vi "configure operation.vi"(7 "tag bus configurable plugin module configuration":refnum<class "Modbus Slave configuration.lvclass">, 8 "error in":errorcluster, 10 "line item in":T2, 11 "engine configuration":refnum<class "engine configuration.lvclass">) -> (0 "error out":errorcluster, 1 "success":bool, 2 "line item out":T2, 5 "changed":bool)   [LabVIEW 2013, in "Modbus Slave editor node.lvclass"]
doc: "Platypus Framework 1.0.1.65\nNI Systems Engineering - National Instruments"
uses:
  Modbus Slave editor node.lvclass
  permissions.ctl
  table line.ctl
  module/module channel/Modbus Module Channel.lvclass
  <vilib>/NI/Module Execution Interface/Engine Configuration/engine configuration.lvclass
  module/configuration/Modbus Slave configuration.lvclass
  module/module channel/data bank type.ctl
  <vilib>/NI/Tag Bus Module Framework/channel/TBM channel.lvclass/TBM channel.ctl
  module/module channel/Modbus Module Channel.lvclass/Modbus Module Channel.ctl
  <vilib>/NI/Tag Bus/tag/tag descriptor.lvclass/tag descriptor.ctl
  <vilib>/NI/Configuration Framework/serializable configuration/NISE_CEF_serializable configuration.lvclass/NISE_CEF_serializable configuration.ctl
  <vilib>/NI/Configuration Framework/serializable configuration/NISE_CEF_serializable configuration.lvclass
  <vilib>/NI/Tag Bus/tag/Data Type.ctl
  <vilib>/NI/Tag Bus Module Framework/channel/Read channel classification.vi
  module/module channel/Read modbus type.vi
  module/module channel/Read starting address.vi
  module/module channel/Read subindex (bool).vi
  <vilib>/NI/Tag Bus/tag/read data type.vi
  <vilib>/NI/Configuration Framework/serializable configuration/Read UID.vi
  <vilib>/NI/Tag Bus/tag/write data type.vi
  <vilib>/NI/Tag Bus Module Framework/channel/Write channel classification.vi
  module/module channel/Write modbus type.vi
  module/module channel/Write starting address.vi
  module/module channel/Write subindex (bool).vi
  <vilib>/NI/Tag Bus/tag/write tag name.vi
  <vilib>/NI/Tag Bus/tag/tag descriptor.lvclass
panel:
  in  "Channel Name":string
  out "Alias":string
  out "issues":string
  in  "Tag":i32(listbox)
  in  "Type":i32(listbox)
  in  "Bit":i32 min=0 max=15 step=1
  in  "Address (0 index)":i32
  in  "modbus bank":T1
  in  "cancel":bool
  in  "ok":bool
  in  "Access Type":T3
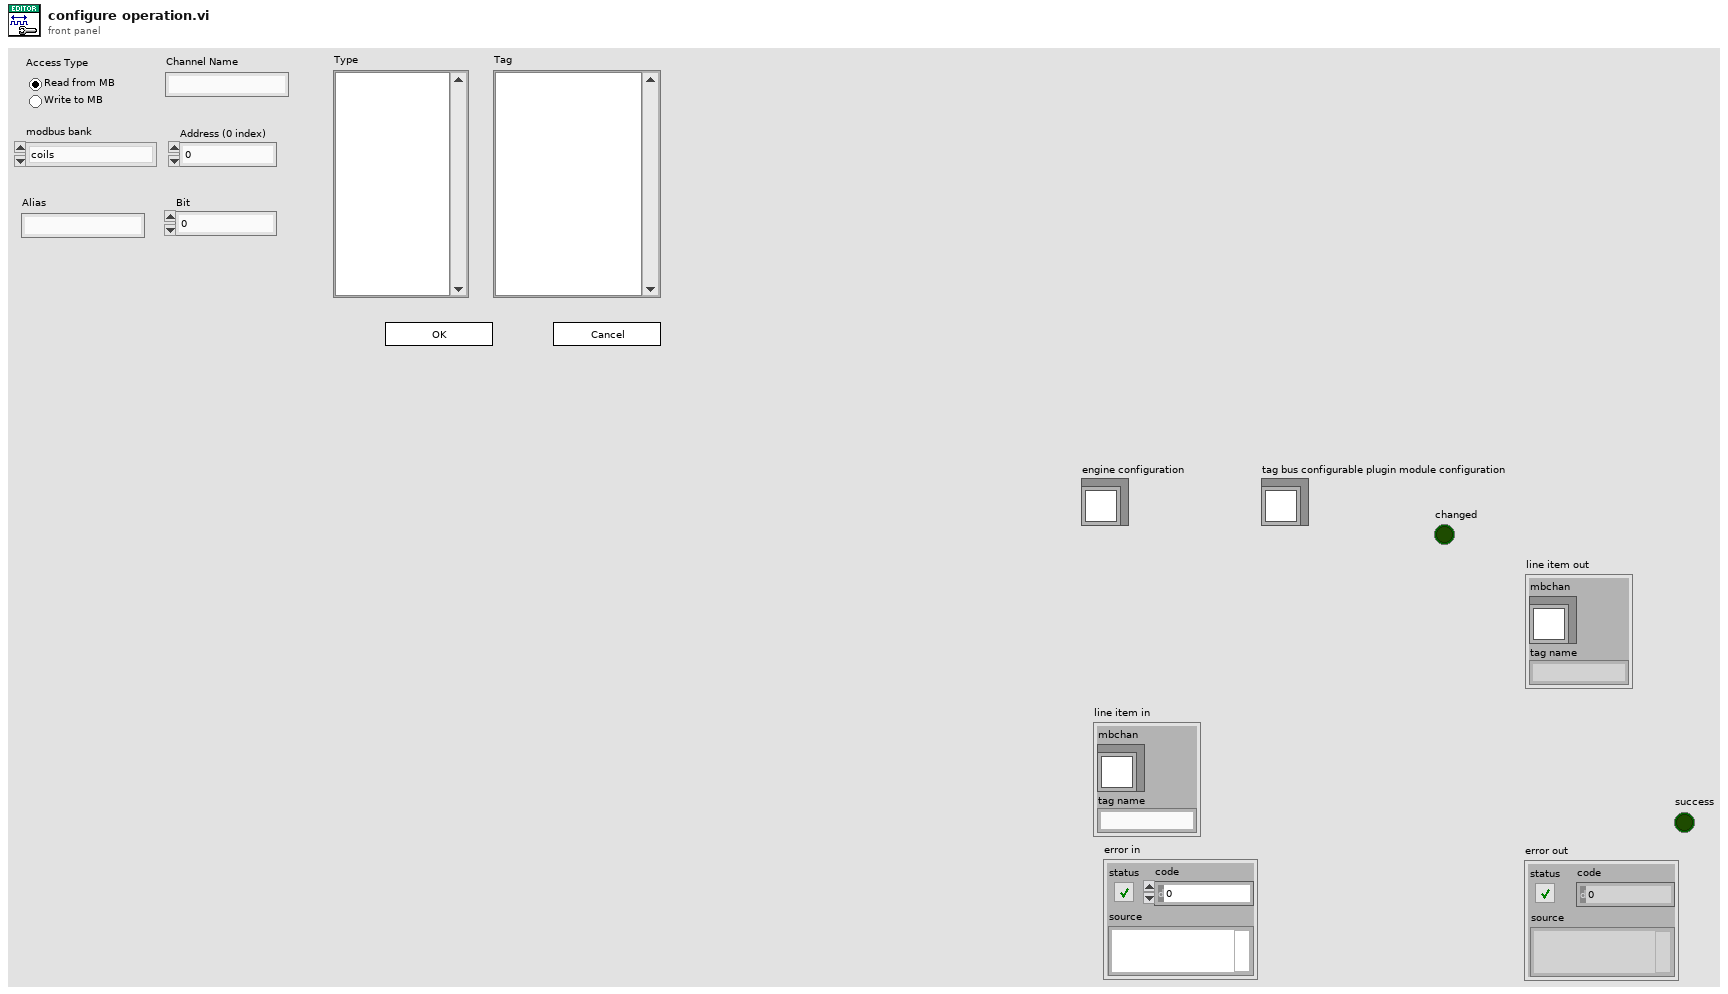
[diagram p1: front panel]
types:
  T1 = typedef "Modbus Module Channel.lvclass/data bank type.ctl" = enum16{"coils", "discrete inputs", "input registers", "holding registers"}
  T2 = typedef "Modbus Slave editor node.lvclass/table line.ctl" = cluster{"mbchan":refnum<class "Modbus Module Channel.lvclass">, "tag name":string}
  T3 = typedef "Modbus Slave editor node.lvclass/permissions.ctl" = enum32{"Read from MB", "Write to MB"}
  T4 = enum32{"Invalid", "Standard", "Closed", "Hidden", "Minimized", "Maximized"}
  T5 = enum32{"Invalid", "Default", "Floating", "Floating/Auto-Hide", "Modal"}
  T6 = enum8{"Enabled", "Disabled", "Disabled and Grayed Out"}
  T7 = typedef "tag bus.lvlib/tag descriptor.lvclass/Data Type.ctl" = enum16{"Double", "Single", "I64", "I32", "I16", "I8", "U64", "U32", "U16", "U8", "Boolean", "String", "Array of Double", "Array of Single", "Array of I64", "Array of I32", "Array of I16", "Array of I8", "Array of U64", "Array of U32", "Array of U16", "Array of U8", "Array of Boolean", "Array of String"}
  T8 = enum32{"invalid app kind", "Development System", "Run Time System", "Student Edition", "Embedded LabVIEW", "Evaluation", "Custom"}
  T9 = typedef "TBM channel.lvclass/channel classification.ctl" = enum16{"input data", "output data", "processing parameter", "processing result"}
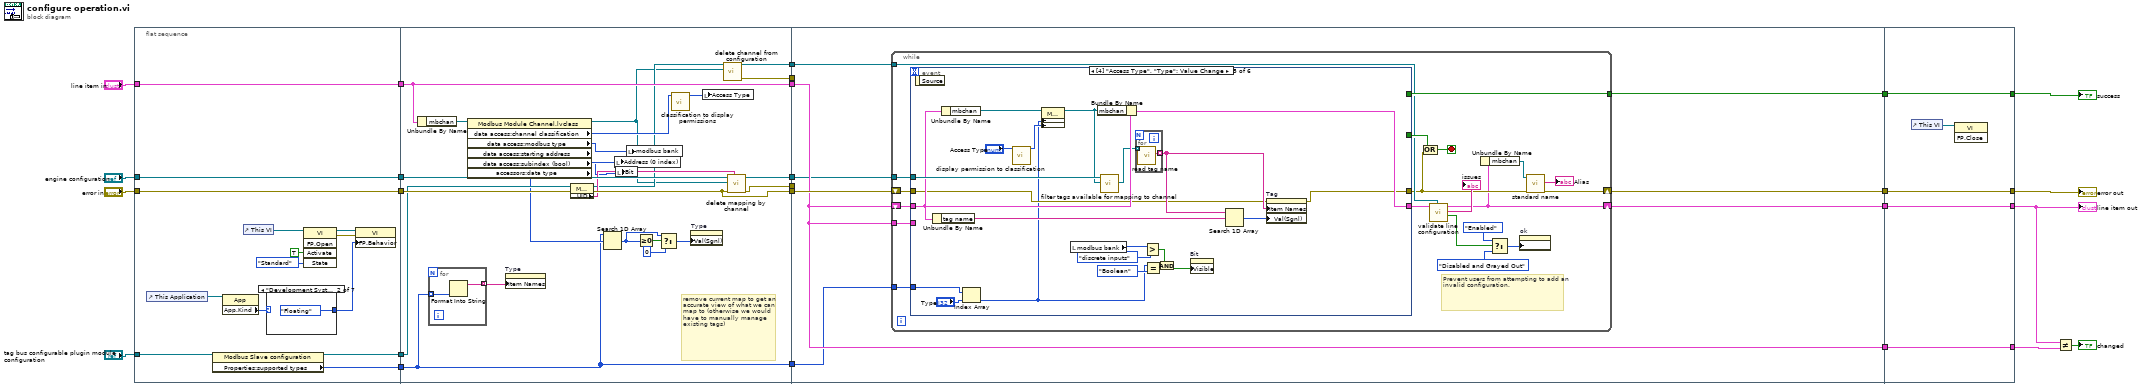
[diagram p0: block diagram]
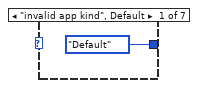
[diagram p2: hidden frame]
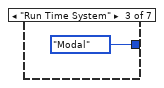
[diagram p3: hidden frame]
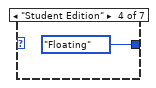
[diagram p4: hidden frame]
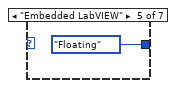
[diagram p5: hidden frame]
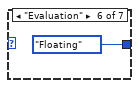
[diagram p6: hidden frame]
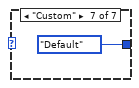
[diagram p7: hidden frame]
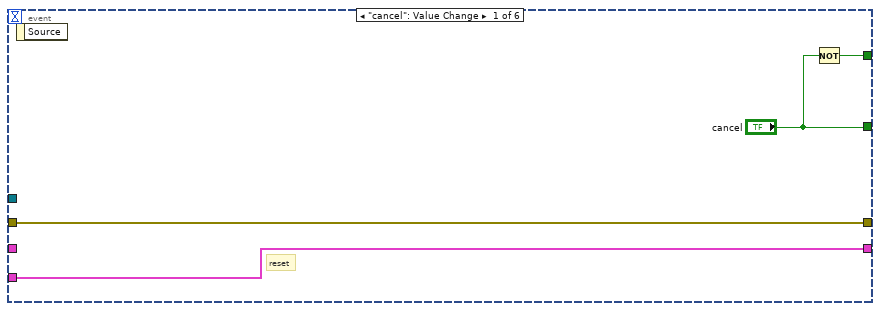
[diagram p8: hidden frame]
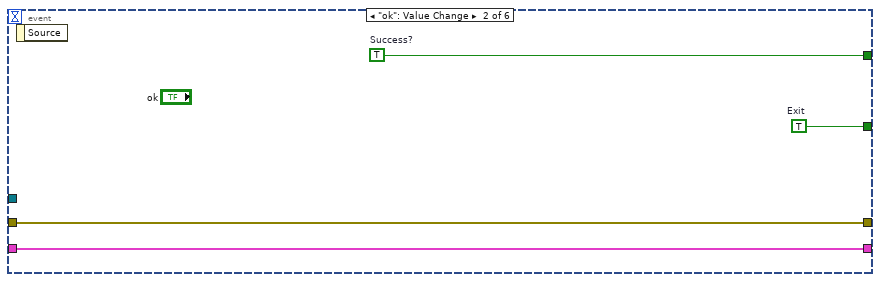
[diagram p9: hidden frame]
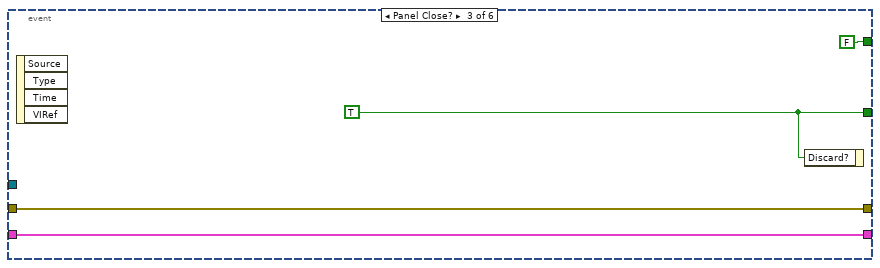
[diagram p10: hidden frame]
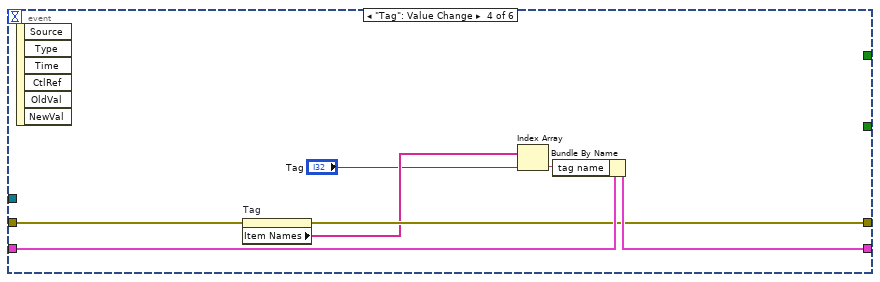
[diagram p11: hidden frame]
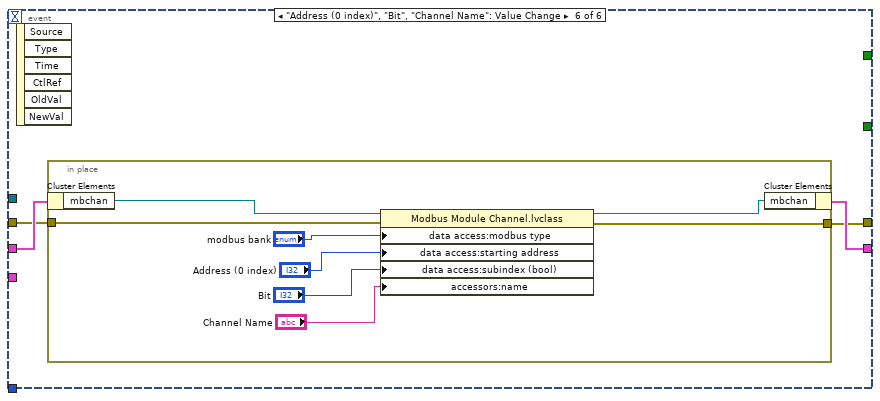
[diagram p12: hidden frame]
diagram:
  n1 = flat-sequence {
    tunnel: "line item in" -> [w38]
    tunnel: "error in" -> [w39]
    tunnel: [w39] -> w14
    tunnel: [w38] -> w13
    tunnel: [w29] -> w10
    tunnel: "engine configuration" -> [w29]
    tunnel: [w27] -> w8
    tunnel: "tag bus configurable plugin module configuration" -> [w28]
    tunnel: [w26] -> w4
    tunnel: w14 -> [w64]
    tunnel: w13 -> [w68]
    tunnel: [w68] -> w12
    tunnel: [w66] -> w11
    tunnel: w10 -> [w67]
    tunnel: w8 -> [w62]
    tunnel: [w63] -> w6
    tunnel: [w65] -> w5
    tunnel: w4 -> [w52]
    tunnel: [w52] -> w3
    tunnel: [w49] -> w2
    tunnel: [w48] -> w1
    tunnel: [w80] -> w18
    tunnel: [w79] -> w17
    tunnel: [w75] -> w16
    tunnel: [w78] -> w15
    tunnel: w12 -> [w78]
    tunnel: w11 -> [w77]
    tunnel: w6 -> [w81]
    tunnel: w5 -> [_]
    tunnel: w3 -> [w74]
    tunnel: w2 -> [w76]
    tunnel: w1 -> [_]
    tunnel: [w158] -> w19
    tunnel: [w159] -> w22
    tunnel: [w160] -> w23
    tunnel: [w161] -> w24
    tunnel: w18 -> [w161]
    tunnel: w17 -> [w160]
    tunnel: w16 -> [w159]
    tunnel: w15 -> [w158]
    frame #0 {
      n2 = control-ref of="This Application"() -> (w32:refnum<vi>)
      n3 = property class="Modbus Slave configuration"(reference=w28) -> (reference out=w27:refnum<class "Modbus Slave configuration.lvclass">, "Properties:supported types"=w26:T7[])  [unwired: 1 in, 1 out]
      n4 = property class="App"(reference=w32) -> ("App.Kind"=w31:T8)  [unwired: 1 in, 2 out]
      n5 = control-ref of="This VI"() -> (w33:refnum<vi>)
      n6 = case shown="\"Development System\"" w31 {
        tunnel: [T5."Default" ("Front Panel Window:Behavior") T5."Floating" ("Front Panel Window:Behavior") T5."Modal" ("Front Panel Window:Behavior") T5."Floating" ("Front Panel Window:Behavior") T5."Floating" ("Front Panel Window:Behavior") T5."Floating" ("Front Panel Window:Behavior") T5."Default" ("Front Panel Window:Behavior")] -> w30
        frame "invalid app kind", Default {
        }
        frame "Development System" {
        }
        frame "Run Time System" {
        }
        frame "Student Edition" {
        }
        frame "Embedded LabVIEW" {
        }
        frame "Evaluation" {
        }
        frame "Custom" {
        }
      }
      n7 = invoke class="VI" method="FP.Open"(reference=w33, "Activate"=TRUE ("Activate?"), "State"=T4."Standard") -> (reference out=w36:refnum<vi>, error out=w37:errorcluster)  [unwired: 2 in, 3 out]
      n8 = property class="VI"(reference=w36, error in=w37, "FP.Behavior"=w30) -> ()  [unwired: 2 out]
    }
    frame #1 {
      # "remove current map to get an accurate view of what we can map to (otherwise we would have to manually manage existing tags)"
      n9 = Unbundle By Name(w68) -> ("mbchan"=w70:refnum<class "Modbus Module Channel.lvclass">)
      n10 = for {
        tunnel: w52 -> [w73] mode=indexing
        tunnel: [w72] -> w51 mode=indexing
        n11 = Format Into String(w73) -> (resulting string=w72:string)  [unwired: 3 in, 1 out]
      }
      n12 = property class="Modbus Module Channel.lvclass"(reference=w70) -> (reference out=w47:refnum<class "Modbus Module Channel.lvclass">, "data access:channel classification"=w71:T9, "data access:modbus type"=w60:T1, "data access:starting address"=w59:u16, "data access:subindex (bool)"=w58:i32, "accessors:data type"=w57:T7)  [unwired: 1 in, 1 out]
      n13 = property on="Type" class="LstBox (strict)"("Item Names"=w51) -> ()  [unwired: 2 in, 2 out]
      n14 = property class="Modbus Slave configuration"(reference=w62, error in=w64) -> (reference out=w50:refnum<class "Modbus Slave configuration.lvclass">, error out=w63:errorcluster, "Properties:UID"=w61:string)
      n15 = Search 1D Array(1D array=w52, element=w57) -> (index of element=w54:i32)  [unwired: 1 in]
      n16 = local write "Address (0 index)"(w59) -> ()
      n17 = local write "Bit"(w58) -> ()
      n18 = local write "modbus bank"(w60) -> ()
      n19 = Greater Or Equal To 0?(x=w54) -> (x >= 0?=w56:bool)
      n20 = Select(t=w54, s=w56, f=0) -> (s? t:f=w55:i32)
      n21 = call "classification to display permissions.vi"("channel classification"=w71) -> ("permissions"=w69:T3)  [unwired: 10 in]
      n22 = property on="Type" class="LstBox (strict)"("Val(Sgnl)"=w55) -> ()  [unwired: 2 in, 2 out]
      n23 = local write "Access Type"(w69) -> ()
      n24 = call "delete channel from configuration.vi"("Modbus Module Channel.lvclass"=w47, "Modbus Slave configuration in"=w50) -> ("error out"=w48:errorcluster, "Modbus Slave configuration out"=w49:refnum<class "Modbus Slave configuration.lvclass">)  [unwired: 8 in]
      n25 = call <vilib>:"delete mapping by channel.vi"("owner ID"=w61, "error in"=w63, "channel"=w47, "engine configuration in"=w67) -> ("error out"=w65:errorcluster, "engine configuration out"=w66:refnum<class "engine configuration.lvclass">)  [unwired: 6 in]
    }
    frame #2 {
      n26 = while {
        shift-right: [w86] -> w79
        shift-left: w81 -> [w100]
        tunnel: [w99] -> w80
        shift-right: [w84] -> w75
        shift-left: w78 -> [w96]
        tunnel: w78 -> [w95]
        tunnel: w77 -> [w101]
        tunnel: w76 -> [w89]
        tunnel: w74 -> [w88]
        stop <- w97 stop-if-true
        # "Prevent users from attempting to add an invalid configuration."
        n27 = event shown="[4] \"Access Type\", \"Type\": Value Change" {
          selector: _ -> [_ _ _ _ _ _]
          dyn-events: _ -> [_ _ _ _ _ _]
          timeout: _ -> [_ _ _ _ _ _]
          tunnel: w101 -> [_ _ _ _ w139 _]
          tunnel: w100 -> [w105 w109 w113 w117 w125 w146]
          tunnel: [w105 w109 w113 w116 w124 w145] -> w85
          tunnel: [w104 w106 FALSE _ _ _] -> w99
          tunnel: ["cancel" w107 w111 _ _ _] -> w98
          tunnel: w96 -> [_ w108 w110 w120 w137 w148]
          tunnel: [w102 w108 w110 w119 w128 w147] -> w94
          tunnel: w95 -> [w102 _ _ _ _ _]
          tunnel: w88 -> [_ _ _ _ w122 _]
          event "cancel": Value Change {
            # "reset"
            n28 = event-data() -> ()  [unwired: 1 in, 1 out]
            n29 = Not(x="cancel") -> (.not. x?=w104:bool)
          }
          event "ok": Value Change {
            w106 = TRUE  # Success?
            w107 = TRUE  # Exit
            n30 = event-data() -> ()  [unwired: 1 in, 1 out]
          }
          event Panel Close? {
            w111 = TRUE ("cancel")
            n31 = event-data() -> ()  [unwired: 1 in, 4 out]
            n32 = event-data("Discard?"=w111) -> ()  [unwired: 1 in, 1 out]
          }
          event "Tag": Value Change {
            n33 = event-data() -> ()  [unwired: 1 in, 6 out]
            n34 = property on="Tag" class="LstBox (strict)"(error in=w117) -> (error out=w116:errorcluster, "Item Names"=w115:string[])  [unwired: 1 in, 1 out]
            n35 = Index Array(array=w115, index="Tag") -> (element=w118:string)
            n36 = Bundle By Name(cluster=w120, "tag name"=w118) -> (w119:T2)
          }
          event "Type": Value Change {
            n37 = event-data() -> ()  [unwired: 1 in, 1 out]
            n38 = Unbundle By Name(w137) -> ("tag name"=w129:string)
            n39 = Unbundle By Name(w137) -> ("mbchan"=w141:refnum<class "Modbus Module Channel.lvclass">)
            n40 = Index Array(array=w122, index="Type") -> (element=w121:T7)
            n41 = call "display permission to classification.vi"("display permissions"="Access Type") -> ("channel classification"=w140:T9)  [unwired: 10 in]
            n42 = property class="Modbus Module Channel.lvclass"(reference=w141, "accessors:data type"=w121, "data access:channel classification"=w140) -> (reference out=w138:refnum<class "Modbus Module Channel.lvclass">)  [unwired: 1 in, 1 out]
            n43 = local read "modbus bank"() -> (w133:T1)
            n44 = Bundle By Name(cluster=w137, "mbchan"=w138) -> (w128:T2)
            n45 = call <vilib>:"filter tags available for mapping to channel.vi"("channel to map to"=w138, "engine configuration in"=w139) -> ("filtered tags"=w136:refnum<class "tag descriptor.lvclass">[])  [unwired: 8 in, 1 out]
            n46 = for {
              tunnel: w136 -> [w144] mode=indexing
              tunnel: [w143] -> w126 mode=indexing
              n47 = call <vilib>:"read tag name.vi"("system tag in"=w144) -> ("name"=w143:string)  [unwired: 8 in, 2 out]
            }
            n48 = Greater?(x=w133, y=data_bank_type."discrete inputs") -> (0:w130:bool)
            n49 = Equal?(x=w121, y=Data_Type."Boolean") -> (x = y?=w134:bool)
            n50 = And(x=w130, y=w134) -> (x .and. y?=w131:bool)
            n51 = property on="Bit" class="DigNum (strict)"("Visible"=w131) -> ()  [unwired: 2 in, 2 out]
            n52 = Search 1D Array(1D array=w126, element=w129) -> (index of element=w127:i32)  [unwired: 1 in]
            n53 = property on="Tag" class="LstBox (strict)"(error in=w125, "Item Names"=w126, "Val(Sgnl)"=w127) -> (error out=w124:errorcluster)  [unwired: 1 in, 1 out]
          }
          event "Address (0 index)", "Bit", "Channel Name": Value Change {
            n54 = event-data() -> ()  [unwired: 1 in, 6 out]
            n55 = in-place {
              in-place-border: w146 -> [w156]
              in-place-border: [w150] -> w145
              n56 = in-place-cluster #1(w148) -> ("mbchan"=w155:refnum<class "Modbus Module Channel.lvclass">)
              n57 = property class="Modbus Module Channel.lvclass"(reference=w155, error in=w156, "data access:modbus type"="modbus bank", "data access:starting address"="Address (0 index)", "data access:subindex (bool)"="Bit", "accessors:name"="Channel Name") -> (reference out=w151:refnum<class "Modbus Module Channel.lvclass">, error out=w150:errorcluster)
              n58 = in-place-cluster #1("mbchan"=w151) -> (w147:T2)
            }
          }
        }
        n59 = Compound Arithmetic op=OR(w98, w85) -> (w97:bool)
        n60 = call "validate line configuration.vi"("modbus"=w89, "line in"=w94) -> ("valid?"=w93:bool, "issues"=→"issues":string, "line out"=w84:T2)  [unwired: 7 in]
        n61 = Unbundle By Name(w84) -> ("mbchan"=w83:refnum<class "Modbus Module Channel.lvclass">)
        n62 = Select(t=T6."Enabled" ("Disabled"), s=w93, f=T6."Disabled and Grayed Out") -> (s? t:f=w90:T6)
        n63 = property on="ok" class="Bool"("DisabledEnum"=w90) -> ()  [unwired: 2 in, 2 out]
        n64 = call "standard name.vi"("error in"=w85, "Modbus Module Channel in"=w83) -> ("error out"=w86:errorcluster, "standard name"=→"Alias":string)  [unwired: 7 in, 1 out]
      }
    }
    frame #3 {
      n65 = control-ref of="This VI"() -> (w157:refnum<vi>)
      n66 = invoke class="VI" method="FP.Close"(reference=w157) -> ()  [unwired: 2 in, 3 out]
    }
  }
  n67 = Not Equal?(x=w22, y=w19) -> (x != y?=→"changed":bool)
  "error out" <- w23
  "success" <- w24
  "line item out" <- w22
